vi "Vision Processing.vi"(4 "error in (no error)":errorcluster, 7 "Image Size":T1=enum."320x240") -> ()   [LabVIEW 2017]
doc: "This VI runs in parallel to other tasks. It gets images from the camera, processes them for color or shape and use that information to affect robot behavior."
uses:
  <vilib>/Rock Robotics/WPI/Camera/WPI_CameraImageSize.ctl
  <vilib>/Rock Robotics/WPI/Camera/WPI_CameraExposure Values.ctl
  Robot Global Data.vi
  <vilib>/Rock Robotics/WPI/Camera/WPI_CameraFrameRate.ctl
  <vilib>/Rock Robotics/WPI/Camera/WPI_CameraWhite Balance Values.ctl
panel:
  in  "Image Size 3":T1=enum."320x240"
  in  "Image Size 2":T1=enum."320x240"
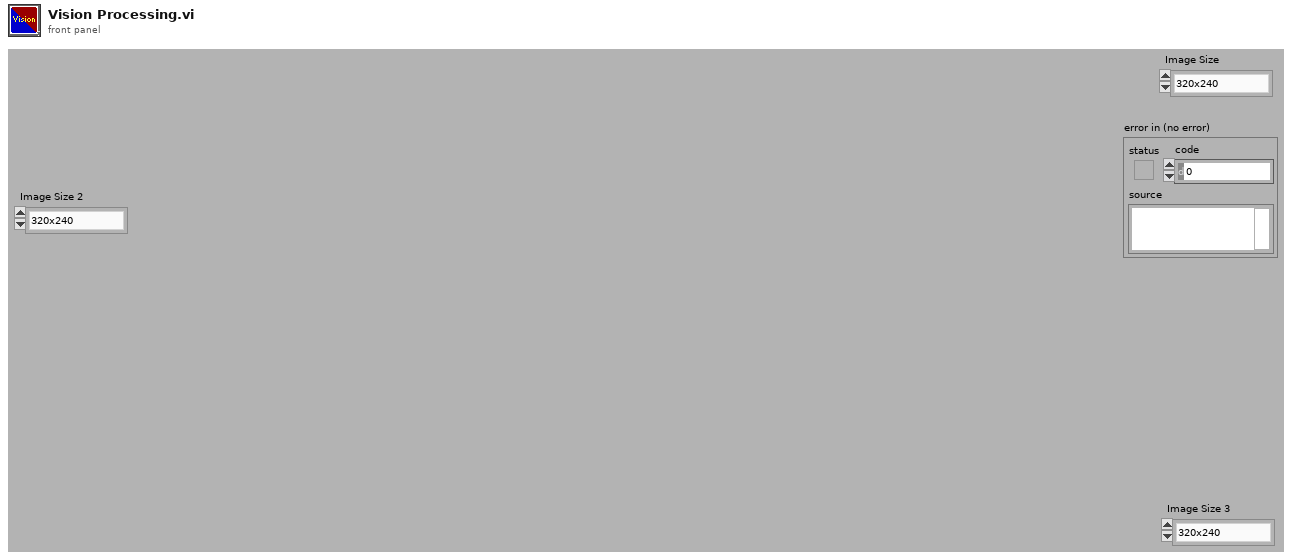
[diagram p1: front panel]
types:
  T1 = typedef "WPI_CameraImageSize.ctl" = enum16{"640x480", "320x240", "160x120", "Custom"}
  T2 = typedef "WPI_CameraExposure Values.ctl" = enum16{"Auto", "Flicker-free 50 Hz", "Flicker-free 60 Hz", "Hold current", "Custom"}
  T3 = typedef "Image Type" = u32
  T4 = typedef "WPI_CameraFrameRate.ctl" = u32
  T5 = typedef "WPI_CameraWhite Balance Values.ctl" = enum16{"Auto", "Fixed indoor", "Fixed outdoor 1", "Fixed outdoor 2", "Fixed fluorescent 1", "Fixed fluorescent 2", "Hold current", "Custom"}
  T6 = typedef "WPI_CameraDevRef.ctl" = cluster{"Camera Address":string, "CameraStatus":errorcluster}
  T7 = typedef "IMAQ Image.ctl" = refnum<image>
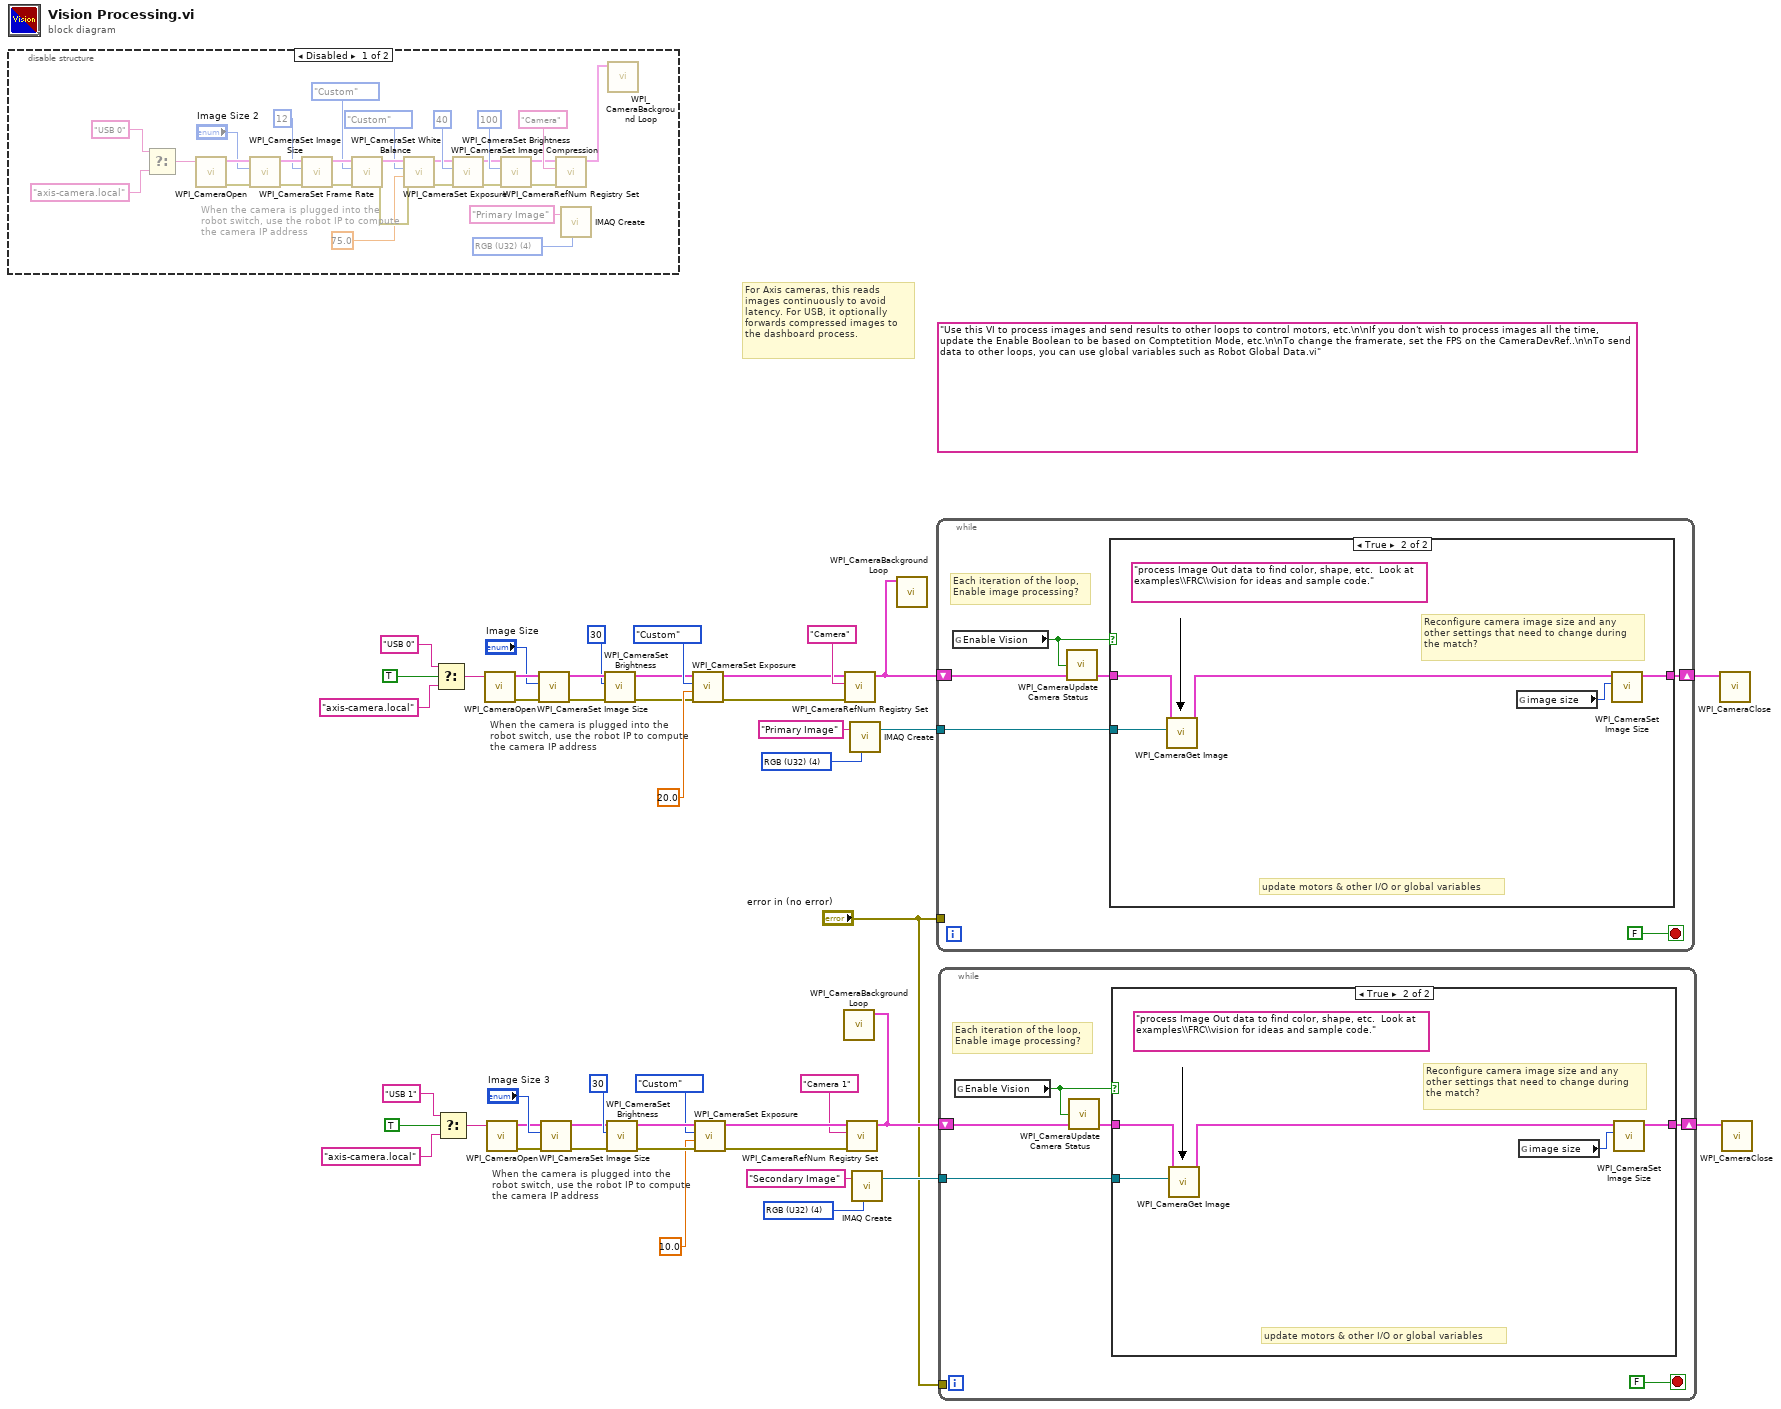
[diagram p0: block diagram]
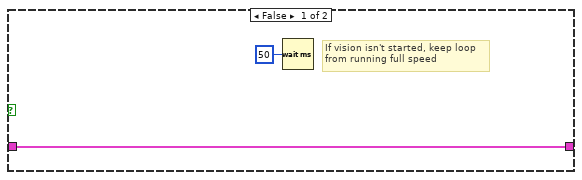
[diagram p2: hidden frame]
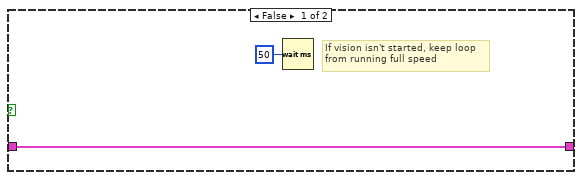
[diagram p4: hidden frame]
diagram:
  w2 = T3 4 items=["Grayscale (U8)", "Grayscale (I16)", "Grayscale (SGL)", "Complex (CSG)", "RGB (U32)", "HSL (U32)", "RGB (U64)"] ("Image Type")
  (unwired) "Use this VI to process images and send results to other loops to control motors, etc.\n\nIf you don't wish to process images all the time, update the Enable Boolean to be based on Comptetition Mode, etc.\n\nTo change the framerate, set the FPS on the CameraDevRef..\n\nTo send data to other loops, you can use global variables such as Robot Global Data.vi"
  w45 = T3 4 items=["Grayscale (U8)", "Grayscale (I16)", "Grayscale (SGL)", "Complex (CSG)", "RGB (U32)", "HSL (U32)", "RGB (U64)"] ("Image Type")
  # "When the camera is plugged into the\nrobot switch, use the robot IP to compute\nthe camera IP address"
  # "When the camera is plugged into the\nrobot switch, use the robot IP to compute\nthe camera IP address"
  # "For Axis cameras, this reads\nimages continuously to avoid\nlatency. For USB, it optionally\nforwards compressed images to\nthe dashboard process."
  n1 = disable-structure shown="Disabled" {
    frame Disabled {
      w75 = T3 4 items=["Grayscale (U8)", "Grayscale (I16)", "Grayscale (SGL)", "Complex (CSG)", "RGB (U32)", "HSL (U32)", "RGB (U64)"] ("Image Type")
      # "When the camera is plugged into the\nrobot switch, use the robot IP to compute\nthe camera IP address"
      n2 = Select(t="USB 0" ("format string"), f="axis-camera.local" ("format string")) -> (s=w49:bool, s? t:f=w48:string)
      n3 = call <vilib>:"WPI_CameraOpen.vi"("Camera Address"=w48) -> ("error out"=w63:errorcluster, "CameraDevRef"=w64:T6)  [unwired: 1 in, 8 out]
      n4 = call <vilib>:"WPI_CameraSet Image Size.vi"("error in (no error)"=w63, "Image Size"="Image Size 2", "CameraDevRef"=w64) -> ("error out"=w62:errorcluster, "CameraDevRef Out"=w65:T6)  [unwired: 1 in, 6 out]
      n5 = call <vilib>:"WPI_CameraSet Frame Rate.vi"("error in (no error)"=w62, "Frame Rate (fps)"=T4 12, "CameraDevRef"=w65) -> ("error out"=w61:errorcluster, "CameraDevRef Out"=w67:T6)  [unwired: 7 out]
      n6 = call <vilib>:"WPI_CameraSet White Balance.vi"("error in (no error)"=w61, "White Balance"=WPI_CameraWhite_Balance_Values."Custom", "CameraDevRef"=w67) -> ("error out"=w60:errorcluster, "CameraDevRef Out"=w66:T6)  [unwired: 1 in, 6 out]
      n7 = call <vilib>:"WPI_CameraSet Exposure.vi"("error in (no error)"=w60, "Exposure (%)"=75.0, "Exposure"=WPI_CameraExposure_Values."Custom", "CameraDevRef"=w66) -> ("error out"=w59:errorcluster, "CameraDevRef Out"=w69:T6)  [unwired: 6 out]
      n8 = call <vilib>:"WPI_CameraSet Image Compression.vi"("error in (no error)"=w59, "Compression"=40, "CameraDevRef"=w69) -> ("error out"=w58:errorcluster, "CameraDevRef Out"=w68:T6)  [unwired: 7 out]
      n9 = call <vilib>:"WPI_CameraSet Brightness.vi"("error in (no error)"=w58, "Brightness"=100, "CameraDevRef"=w68) -> ("error out"=w56:errorcluster, "CameraDevRef Out"=w57:T6)  [unwired: 1 in, 6 out]
      n10 = call <vilib>:"WPI_CameraRefNum Registry Set.vi"("error in (no error)"=w56, "refnum name"="Camera", "CameraDevRef"=w57) -> ("CameraDevRef"=w52:T6)  [unwired: 1 in, 7 out]
      n11 = call "IMAQ Create"("Image Name"="Primary Image", "Image Type"=w75) -> ("New Image"=w73:T7)  [unwired: 2 in, 2 out]
      n12 = call <vilib>:"WPI_CameraBackground Loop.vi"("CameraDevRef"=w52) -> ()  [unwired: 11 in]
    }
    frame Enabled {
    }
  }
  n13 = Select(t="USB 0" ("format string"), s=TRUE ("dot notation? (F)"), f="axis-camera.local" ("format string")) -> (s? t:f=w33:string)
  n14 = Select(t="USB 1" ("format string"), s=TRUE ("dot notation? (F)"), f="axis-camera.local" ("format string")) -> (s? t:f=w14:string)
  n15 = call <vilib>:"WPI_CameraOpen.vi"("Camera Address"=w33) -> ("error out"=w40:errorcluster, "CameraDevRef"=w41:T6)  [unwired: 1 in, 8 out]
  n16 = call <vilib>:"WPI_CameraOpen.vi"("Camera Address"=w14) -> ("error out"=w7:errorcluster, "CameraDevRef"=w6:T6)  [unwired: 1 in, 8 out]
  n17 = call <vilib>:"WPI_CameraSet Image Size.vi"("error in (no error)"=w40, "Image Size"="Image Size", "CameraDevRef"=w41) -> ("error out"=w27:errorcluster, "CameraDevRef Out"=w28:T6)  [unwired: 1 in, 6 out]
  n18 = call <vilib>:"WPI_CameraSet Image Size.vi"("error in (no error)"=w7, "Image Size"="Image Size 3", "CameraDevRef"=w6) -> ("error out"=w20:errorcluster, "CameraDevRef Out"=w19:T6)  [unwired: 1 in, 6 out]
  n19 = call <vilib>:"WPI_CameraSet Brightness.vi"("error in (no error)"=w27, "Brightness"=30, "CameraDevRef"=w28) -> ("error out"=w25:errorcluster, "CameraDevRef Out"=w26:T6)  [unwired: 1 in, 6 out]
  n20 = call <vilib>:"WPI_CameraSet Brightness.vi"("error in (no error)"=w20, "Brightness"=30, "CameraDevRef"=w19) -> ("error out"=w22:errorcluster, "CameraDevRef Out"=w21:T6)  [unwired: 1 in, 6 out]
  n21 = call <vilib>:"WPI_CameraSet Exposure.vi"("error in (no error)"=w25, "Exposure (%)"=20.0, "Exposure"=WPI_CameraExposure_Values."Custom", "CameraDevRef"=w26) -> ("error out"=w29:errorcluster, "CameraDevRef Out"=w30:T6)  [unwired: 6 out]
  n22 = call <vilib>:"WPI_CameraSet Exposure.vi"("error in (no error)"=w22, "Exposure (%)"=10.0, "Exposure"=WPI_CameraExposure_Values."Custom", "CameraDevRef"=w21) -> ("error out"=w18:errorcluster, "CameraDevRef Out"=w17:T6)  [unwired: 6 out]
  n23 = call <vilib>:"WPI_CameraRefNum Registry Set.vi"("error in (no error)"=w29, "refnum name"="Camera", "CameraDevRef"=w30) -> ("CameraDevRef"=w38:T6)  [unwired: 1 in, 7 out]
  n24 = call <vilib>:"WPI_CameraRefNum Registry Set.vi"("error in (no error)"=w18, "refnum name"="Camera 1", "CameraDevRef"=w17) -> ("CameraDevRef"=w9:T6)  [unwired: 1 in, 7 out]
  n25 = call <vilib>:"WPI_CameraBackground Loop.vi"("CameraDevRef"=w9) -> ()  [unwired: 11 in]
  n26 = call "IMAQ Create"("Image Name"="Primary Image", "Image Type"=w45) -> ("New Image"=w43:T7)  [unwired: 2 in, 2 out]
  n27 = call "IMAQ Create"("Image Name"="Secondary Image", "Image Type"=w2) -> ("New Image"=w4:T7)  [unwired: 2 in, 2 out]
  n28 = call <vilib>:"WPI_CameraBackground Loop.vi"("CameraDevRef"=w38) -> ()  [unwired: 11 in]
  n29 = while {
    shift-right: [w80] -> w36
    shift-left: w38 -> [w78]
    tunnel: w43 -> [w79]
    tunnel: "error in (no error)" -> [_]
    stop <- FALSE stop-if-true
    # "Each iteration of the loop,\nEnable image processing?"
    n30 = global read "Robot Global Data.vi" "Enable Vision"() -> (w76:bool)
    n31 = call <vilib>:"WPI_CameraUpdate Camera Status.vi"("CameraDevRef In"=w78, "Enable Vision"=w76) -> ("CameraDevRef Out"=w77:T6)  [unwired: 3 in]
    n32 = case shown="True" w76 {
      tunnel: w79 -> [_ w87]
      tunnel: [w83 w88] -> w80
      tunnel: w77 -> [w83 w85]
      frame False {
        # "If vision isn't started, keep loop\nfrom running full speed"
        n33 = Wait (ms)(milliseconds to wait=u32 50) -> ()  [unwired: 1 out]
      }
      frame True {
        (unwired) "process Image Out data to find color, shape, etc.  Look at examples\\FRC\\vision for ideas and sample code."
        # "update motors & other I/O or global variables"
        # "Reconfigure camera image size and any\nother settings that need to change during\nthe match?"
        n34 = call <vilib>:"WPI_CameraGet Image.vi"("Image"=w87, "CameraDevRef"=w85) -> ("CameraDevRef Out"=w84:T6)  [unwired: 1 in, 8 out]
        n35 = global read "Robot Global Data.vi" "image size"() -> (w86:T1)
        n36 = call <vilib>:"WPI_CameraSet Image Size.vi"("Image Size"=w86, "CameraDevRef"=w84) -> ("CameraDevRef Out"=w88:T6)  [unwired: 2 in, 7 out]
      }
    }
  }
  n37 = while {
    shift-right: [w93] -> w11
    shift-left: w9 -> [w91]
    tunnel: w4 -> [w92]
    tunnel: "error in (no error)" -> [_]
    stop <- FALSE stop-if-true
    # "Each iteration of the loop,\nEnable image processing?"
    n38 = global read "Robot Global Data.vi" "Enable Vision"() -> (w89:bool)
    n39 = call <vilib>:"WPI_CameraUpdate Camera Status.vi"("CameraDevRef In"=w91, "Enable Vision"=w89) -> ("CameraDevRef Out"=w90:T6)  [unwired: 3 in]
    n40 = case shown="True" w89 {
      tunnel: w92 -> [_ w100]
      tunnel: [w96 w101] -> w93
      tunnel: w90 -> [w96 w98]
      frame False {
        # "If vision isn't started, keep loop\nfrom running full speed"
        n41 = Wait (ms)(milliseconds to wait=u32 50) -> ()  [unwired: 1 out]
      }
      frame True {
        (unwired) "process Image Out data to find color, shape, etc.  Look at examples\\FRC\\vision for ideas and sample code."
        # "update motors & other I/O or global variables"
        # "Reconfigure camera image size and any\nother settings that need to change during\nthe match?"
        n42 = call <vilib>:"WPI_CameraGet Image.vi"("Image"=w100, "CameraDevRef"=w98) -> ("CameraDevRef Out"=w97:T6)  [unwired: 1 in, 8 out]
        n43 = global read "Robot Global Data.vi" "image size"() -> (w99:T1)
        n44 = call <vilib>:"WPI_CameraSet Image Size.vi"("Image Size"=w99, "CameraDevRef"=w97) -> ("CameraDevRef Out"=w101:T6)  [unwired: 2 in, 7 out]
      }
    }
  }
  n45 = call <vilib>:"WPI_CameraClose.vi"("CameraDevRef"=w36) -> ()  [unwired: 1 in, 10 out]
  n46 = call <vilib>:"WPI_CameraClose.vi"("CameraDevRef"=w11) -> ()  [unwired: 1 in, 10 out]
